vi "ICRA2024最后的ratio控制加轨迹跟踪修改版.vi"() -> ()   [LabVIEW 2018]
doc: "Demonstrates the use of the Network Streams functions to send LED status to the myRIO target."
uses:
  <vilib>/Utility/file.llb/Read Delimited Spreadsheet (string).vi
  <vilib>/ErrorRing/Error Ring.xnode
  <vilib>/vision/NI_Vision_Development_Module.lvlib
panel:
  out "阈值":dbl
  out "ooo":dbl
  out "TT":dbl
  out "与终点距离":sgl
  out "mmm":dbl
  out "期望的ratio":dbl
  out "方向控制量":dbl
  out "速度控制量":dbl
  in  "分裂后的ratio":dbl=3.0
  in  "第二个desiredratio":dbl=7.0
  in  "第一个desiredratio":dbl=3.0
  in  "速度大小":dbl=2.0
  in  "终点纵坐标":dbl=648.0
  in  "终点横坐标":dbl=1450.0
  out "实际纵坐标":sgl[](array[numeric])
  out "实际横坐标":sgl[](array[numeric])
  out "实际纵坐标":sgl
  out "实际横坐标":sgl
  out "方向d1":sgl
  out "轨迹跟踪点数":i32
  out "y":dbl
  out "x":dbl
  out "b":dbl[](array[numeric])
  in  "pp":dbl
  out "与目标点的距离":sgl
  in  "guiji":path=path "D:/lyz/ICRA2024-YuezhenLiu/small_myRIO_Helmholtz - 1111ke777/zgj平滑后的轨迹.txt" caption="call7-8"
  out "ratio误差的绝对值":dbl[](array[numeric])
  in  "pd":dbl=0.1
  out "最终的ratio控制量":dbl
  in  "小p":dbl=1.5
  out "ratio误差的绝对值":dbl
  out "ratio的误差":dbl[](array[numeric])
  out "第二个前馈":dbl
  out "第一个前馈":dbl
  out "后一个ratio误差":dbl
  out "前一个ratio误差":dbl
  out "第一个i":i32
  out "ratio的误差":dbl
  out "裁剪后的二值图":T1(plugin-control)
  in  "布尔":bool
  in  "ribbon磁场开关":bool=TRUE
  out "面积":sgl[](array[numeric])
  out "面积":sgl
  out "数据总":dbl[][](array[numeric])
  out "i":i32[](array[numeric])
  out "aspect ratio":dbl[](array[numeric])
  out "D2":i32[](array[numeric])
  out "D1":i32[](array[numeric])
  out "field ratio":sgl[](array[numeric])
  out "field ratio":sgl=4.0
  out "时间":i32
  in  "打开数据记录":bool
  out "aspect ratio":dbl
  out "D2":i32
  out "D1":i32
  out "二值图":T1(plugin-control)
  in  "Search Rect (entire image)":T2={"Left"=100, "Top"=120, "Right"=2000, "Bottom"=2000, "Rotation"=0.0} {"Rotation" format="%.2f"; "Left" scale=0.0..1024.0; "Right" scale=0.0..1024.0}
  out "备用的椭圆角度":sgl
  in  "Number of Erosion":i32=10
  out "Image 7":T1(plugin-control)
  in  "Acquisition Control::Acquisition Frame Rate":dbl=19.50304412841797 min=1.4211589097976685 max=44.94382095336914
  out "Stopped":bool
  in  "Stop (F) 2":bool caption="Stop (F)"
  out "Objects 2":T3(array[cluster]) {"Aspect Ratio" format="%.2f"; "Orientation" format="%.2f"; "Area" format="%.2f"; "Object Center"."Y" format="%.2f"; "Object Center"."X" format="%.2f"}
  in  "Settings 2":T4={"Objects"=0, "Threshold"=128, "Reject Border"=FALSE, "Fill Holes"=FALSE, "Min Object Size"=FALSE, "Min Size"=20000, "Max Object Size"=FALSE, "Max Size"=100, "Show Search Area"=FALSE, "Show Center"=TRUE, "Show Bounding Box"=TRUE} {"Objects" items=["Bright Objects", "Dark Objects"]; "Threshold" min=1 max=999999999 step=1; "Max Size" min=1 max=999999999 step=1; "Min Size" min=1 max=999999999 step=1}
  in  "Range 2":cluster{"Lower value":sgl, "Upper value":sgl}={"Lower value"=0.0, "Upper value"=230.0} {"Upper value" format="%.2f"; "Lower value" format="%.2f"}
  in  "Pause":bool
  out "Array":dbl[](array[numeric])
  in  "Parameter Settings":T5(tab)=enum."Ribbon Oscillating Field" caption="Field Types"
  in  "fg":dbl
  in  "pg":dbl
  in  "dg":dbl
  in  "Ag":dbl
  in  "AoOF":dbl
  in  "fo":sgl
  in  "do":sgl
  in  "oo":sgl
  in  "po":sgl
  in  "cc":sgl
  in  "pc":sgl
  in  "wc":sgl
  in  "dc":sgl
  in  "Ac":dbl
  in  "pr":sgl
  in  "Ar":dbl=8.0
  in  "wr":sgl=18.0
  in  "dr":sgl
  in  "Dis phase step":dbl
  in  "Dis phase frequency (Hz)":dbl
  in  "Dis tumbling frequency (Hz)":dbl
  in  "Dis strength(mT)":dbl
  in  "Swa strength (mT)":dbl
  in  "Swa frequency (Hz)":dbl
  in  "Swa pitch angle (deg)":dbl
  in  "Swa direction angle (deg)":dbl
  in  "Swa ratio":dbl=1.0
  in  "Pitch Angle (rotating around Constant, deg)":dbl
  in  "Ratio (A/C)":sgl=4.0
  in  "Direction Angle (deg)":sgl
  in  "Pitch Angle (rotating around Origin, deg)":sgl
  in  "Frequency (Hz)":sgl=10.0
  in  "Strength (mT)":dbl=10.0
  in  "Ar 2":dbl=5.0 caption="Ar"
  in  "ratio":sgl=1.0
  in  "运动方向":sgl
  in  "长轴方向":sgl
  in  "wr  2":sgl=8.0
  in  "速度大小":sgl
  out "Numeric 5":i32
  in  "Stop":bool
  out "error out":errorcluster
  in  "Target IP Address":string="172.22.11.2"
  # "Overview: Magnetic field calculation, and send parameters to myRIO\nInstructions:\n1. Verify the value of Target IP Address. Set Visa resource name.\n2. Ensure RT Main.vi is already running. \n3. Run this VI. Set parameters of magnetic field."
  # "Strength (mT)"
  # "Pitch Angle (deg)"
  # "Direction Angle (deg)"
  # "Frequency (Hz)"
  # "Strength (mT)"
  # "Oscilation Frequency (Hz)"
  # "Oscilation Angle (deg)"
  # "Pitch Angle (deg)"
  # "Direction Angle (deg)"
  # "Strength (mT)"
  # "Frequency (Hz)"
  # "Pitch Angle (deg)"
  # "Direction Angle (deg)"
  # "Conical Angle (deg)"
  # "Strength (mT)"
  # "Frequency (Hz)"
  # "Pitch Angle (deg)"
  # "Direction Angle (deg)"
  # "Strength (mT)"
  # "Tumbling Frequency (Hz)"
  # "Phase Frequency (Hz)"
  # "Phase Step"
  # "Strength (mT)"
  # "Frequency (Hz)"
  # "Pitch Angle (deg)"
  # "Direction Angle (deg)"
  # "Ratio"
  # "Strength (mT)"
  # "Frequency (Hz)"
  # "Ratio (A/C)"
  # "Direction Angle (deg)"
  # "Pitch Angle (rotating around Origin, deg)"
  # "Pitch Angle (rotating around Constant, deg)"
  # "Strength (mT)"
  # "Frequency (Hz)"
  # "Pitch Angle  (deg)"
  # "longaxis"
  # "Direction Angle (deg)"
  # "ratio (l/s)"
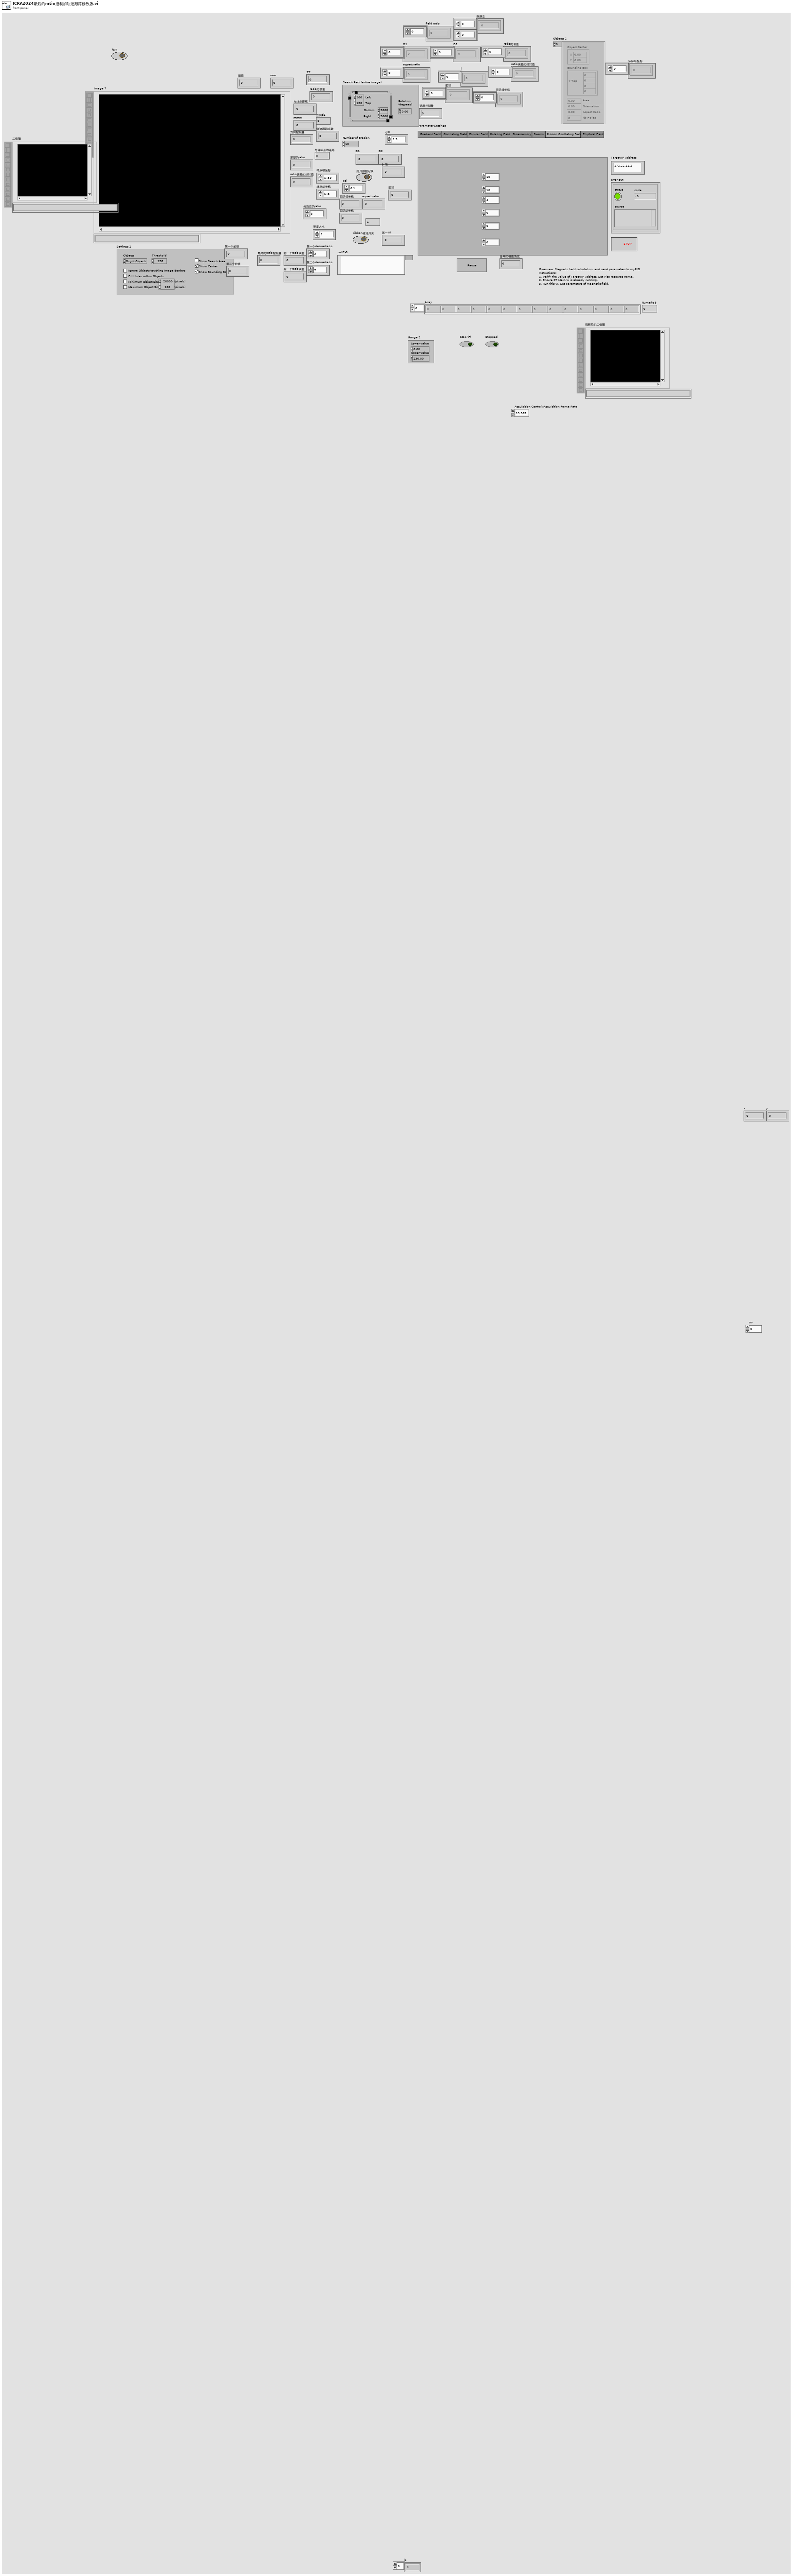
[diagram p1: front panel]
types:
  T1 = typedef "IMAQ Image.ctl" = refnum<image>
  T2 = typedef "IMAQ Rectangle" = cluster{"Left":i32, "Top":i32, "Right":i32, "Bottom":i32, "Rotation":dbl}
  T3 = cluster{"Object Center":cluster{"X":sgl, "Y":sgl}, "Bounding Box":cluster{"X Left":i32, "Y Top":i32, "X Right":i32, "Y Bottom":i32}, "Area":sgl, "Orientation":sgl, "Aspect Ratio":sgl, "Nb Holes":i32}[]
  T4 = cluster{"Objects":u16, "Threshold":i32, "Reject Border":bool, "Fill Holes":bool, "Min Object Size":bool, "Min Size":i32, "Max Object Size":bool, "Max Size":i32, "Show Search Area":bool, "Show Center":bool, "Show Bounding Box":bool}
  T5 = enum32{"Gradient Field ", "Oscillating Field", "Conical Field", "Rotating Field", "Disassembly", "Swarm", "Ribbon Oscillating Field", "Elliptical Field"}
  T6 = typedef "Image Type" = u32
  T7 = cluster{"Objects[0]":cluster{"Object Center":cluster{"X":sgl, "Y":sgl}, "Bounding Box":cluster{"X Left":i32, "Y Top":i32, "X Right":i32, "Y Bottom":i32}, "Area":sgl, "Orientation":sgl, "Aspect Ratio":sgl, "Nb Holes":i32}, "Objects[1]":cluster{"Object Center":cluster{"X":sgl, "Y":sgl}, "Bounding Box":cluster{"X Left":i32, "Y Top":i32, "X Right":i32, "Y Bottom":i32}, "Area":sgl, "Orientation":sgl, "Aspect Ratio":sgl, "Nb Holes":i32}, "Objects[2]":cluster{"Object Center":cluster{"X":sgl, "Y":sgl}, "Bounding Box":cluster{"X Left":i32, "Y Top":i32, "X Right":i32, "Y Bottom":i32}, "Area":sgl, "Orientation":sgl, "Aspect Ratio":sgl, "Nb Holes":i32}, "Objects[3]":cluster{"Object Center":cluster{"X":sgl, "Y":sgl}, "Bounding Box":cluster{"X Left":i32, "Y Top":i32, "X Right":i32, "Y Bottom":i32}, "Area":sgl, "Orientation":sgl, "Aspect Ratio":sgl, "Nb Holes":i32}, "Objects[4]":cluster{"Object Center":cluster{"X":sgl, "Y":sgl}, "Bounding Box":cluster{"X Left":i32, "Y Top":i32, "X Right":i32, "Y Bottom":i32}, "Area":sgl, "Orientation":sgl, "Aspect Ratio":sgl, "Nb Holes":i32}, "Objects[5]":cluster{"Object Center":cluster{"X":sgl, "Y":sgl}, "Bounding Box":cluster{"X Left":i32, "Y Top":i32, "X Right":i32, "Y Bottom":i32}, "Area":sgl, "Orientation":sgl, "Aspect Ratio":sgl, "Nb Holes":i32}, "Objects[6]":cluster{"Object Center":cluster{"X":sgl, "Y":sgl}, "Bounding Box":cluster{"X Left":i32, "Y Top":i32, "X Right":i32, "Y Bottom":i32}, "Area":sgl, "Orientation":sgl, "Aspect Ratio":sgl, "Nb Holes":i32}, "Objects[7]":cluster{"Object Center":cluster{"X":sgl, "Y":sgl}, "Bounding Box":cluster{"X Left":i32, "Y Top":i32, "X Right":i32, "Y Bottom":i32}, "Area":sgl, "Orientation":sgl, "Aspect Ratio":sgl, "Nb Holes":i32}, "Objects[8]":cluster{"Object Center":cluster{"X":sgl, "Y":sgl}, "Bounding Box":cluster{"X Left":i32, "Y Top":i32, "X Right":i32, "Y Bottom":i32}, "Area":sgl, "Orientation":sgl, "Aspect Ratio":sgl, "Nb Holes":i32}}
  T8 = cluster{"Object Center":cluster{"X":sgl, "Y":sgl}, "Bounding Box":cluster{"X Left":i32, "Y Top":i32, "X Right":i32, "Y Bottom":i32}, "Area":sgl, "Orientation":sgl, "Aspect Ratio":sgl, "Nb Holes":i32}
  T9 = cluster{"X Left":i32, "Y Top":i32, "X Right":i32, "Y Bottom":i32}
  T10 = typedef "ROI Descriptor" = cluster{"Global Rectangle":i32[], "Contours":cluster{"ID":enum32{"External", "Internal"}, "Type":u32, "Coordinates":i32[]}[]}
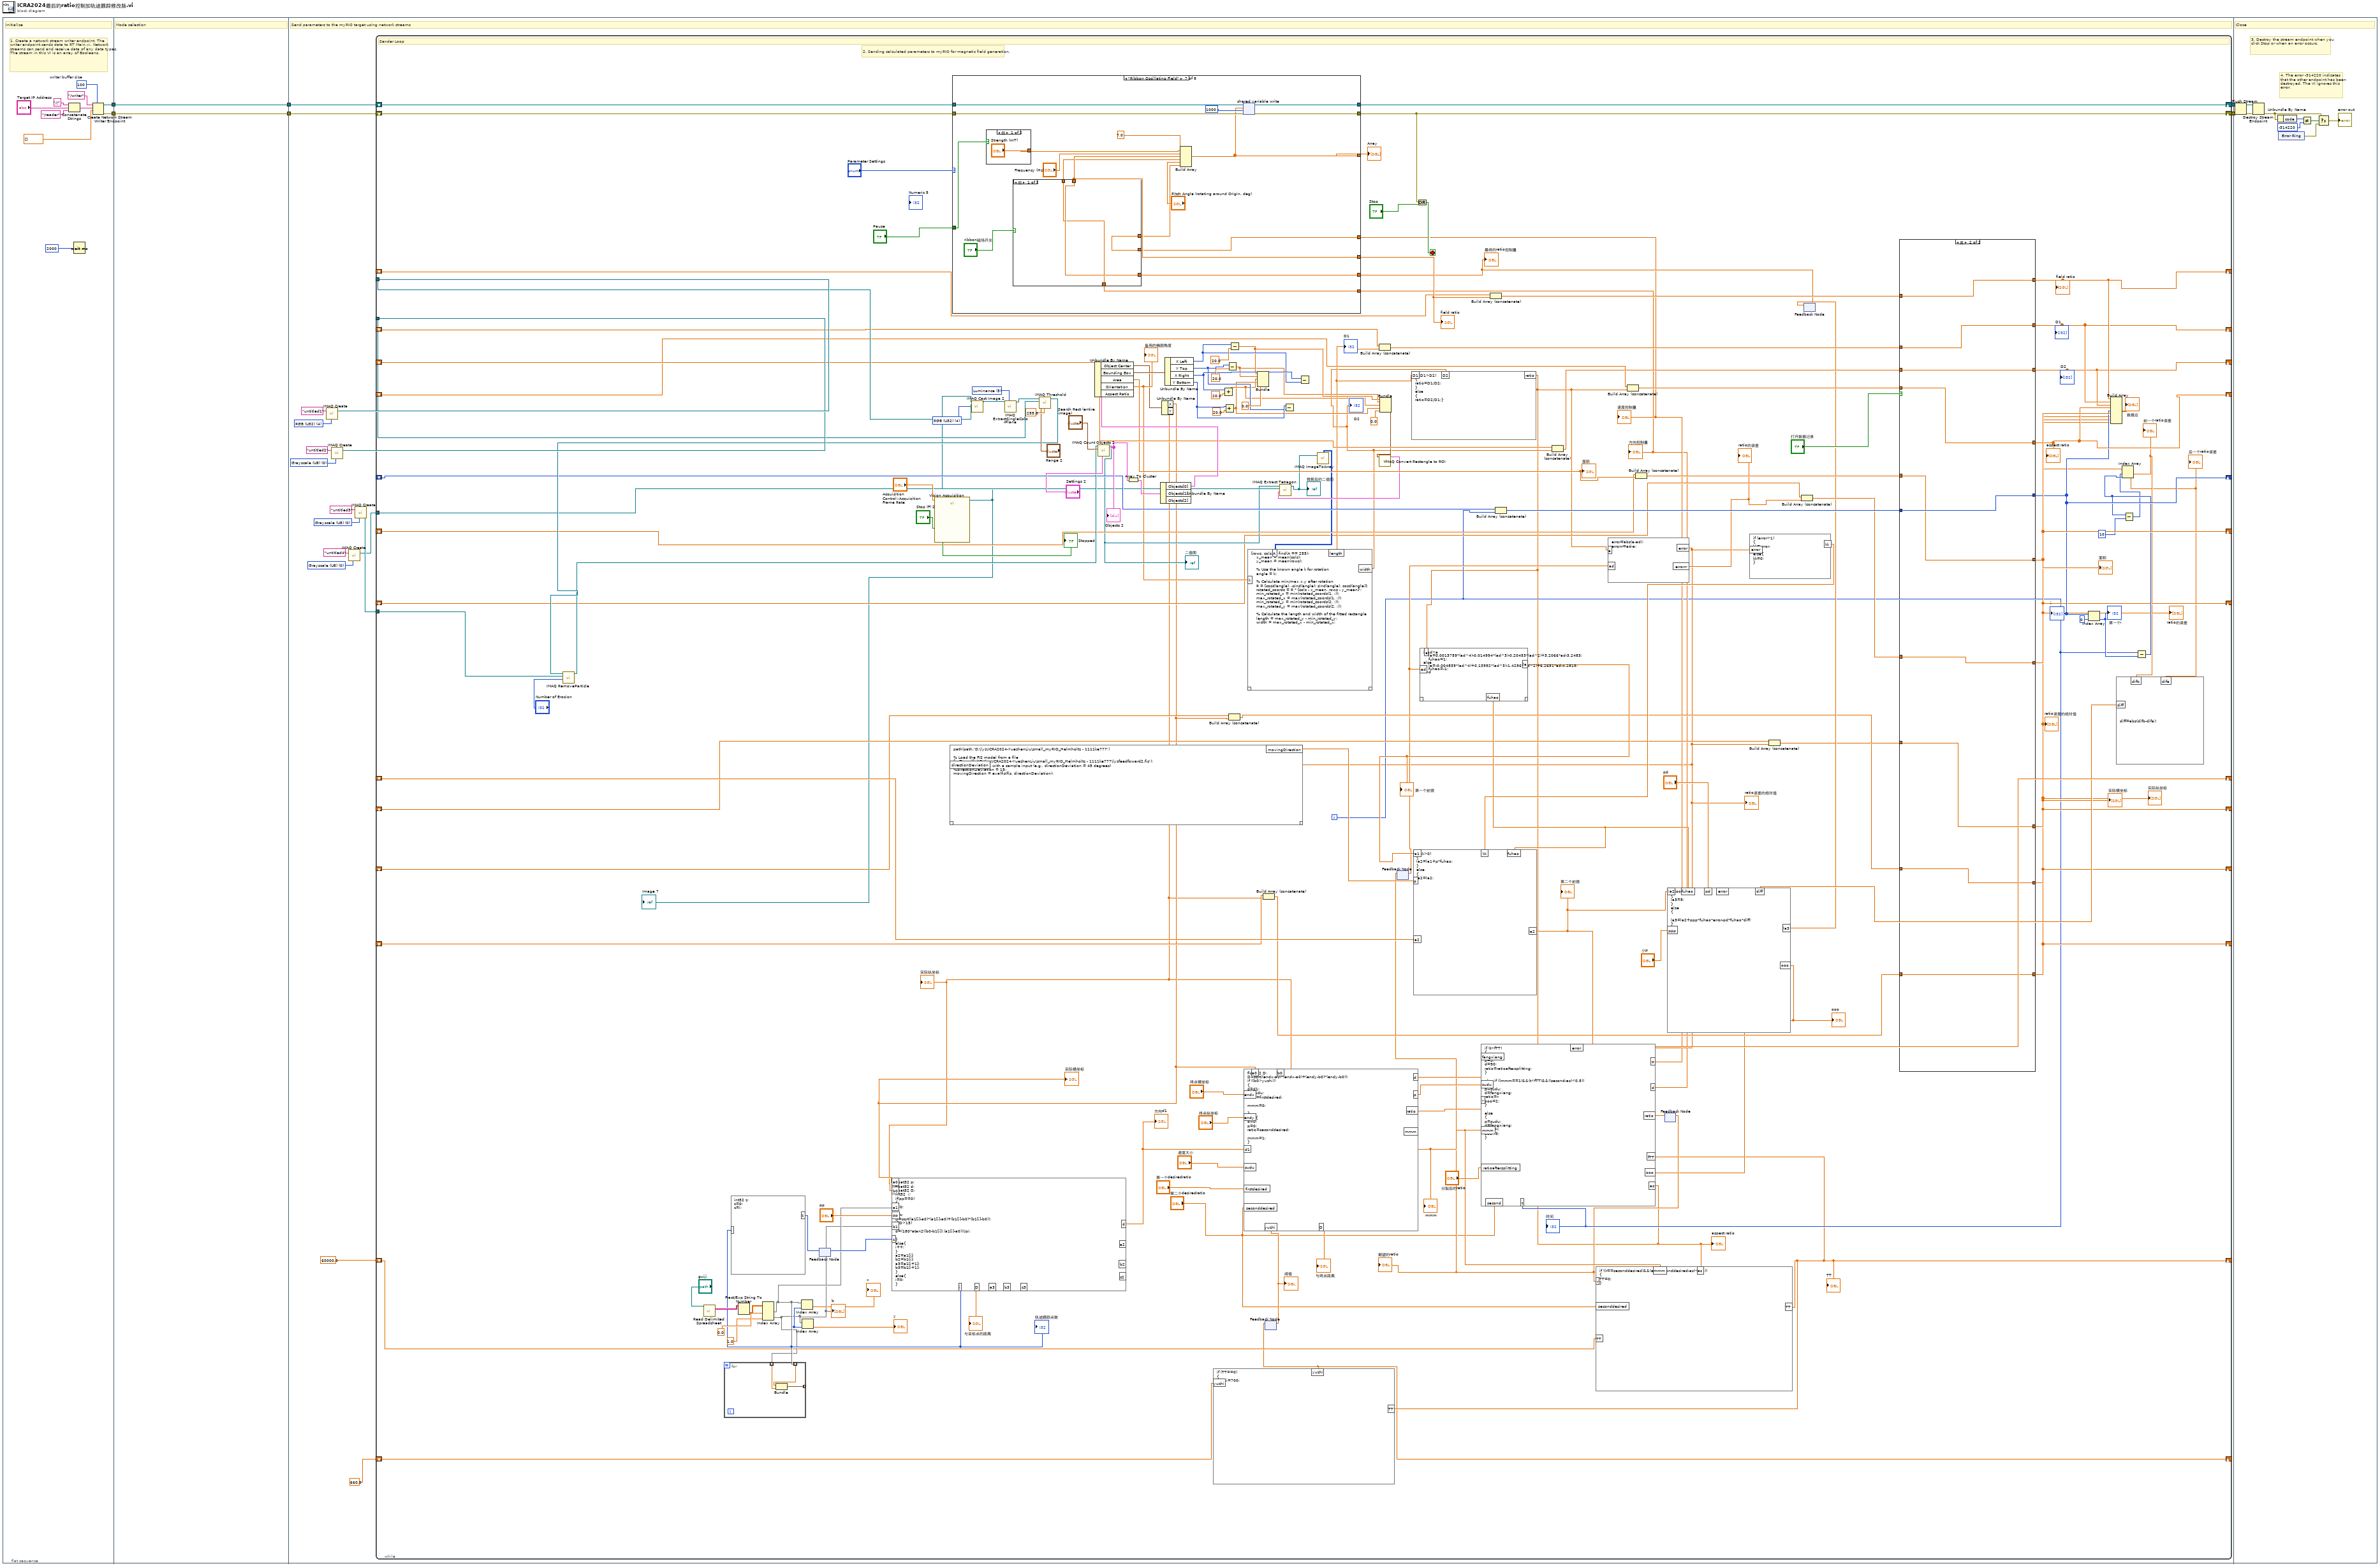
[diagram p0: block diagram]
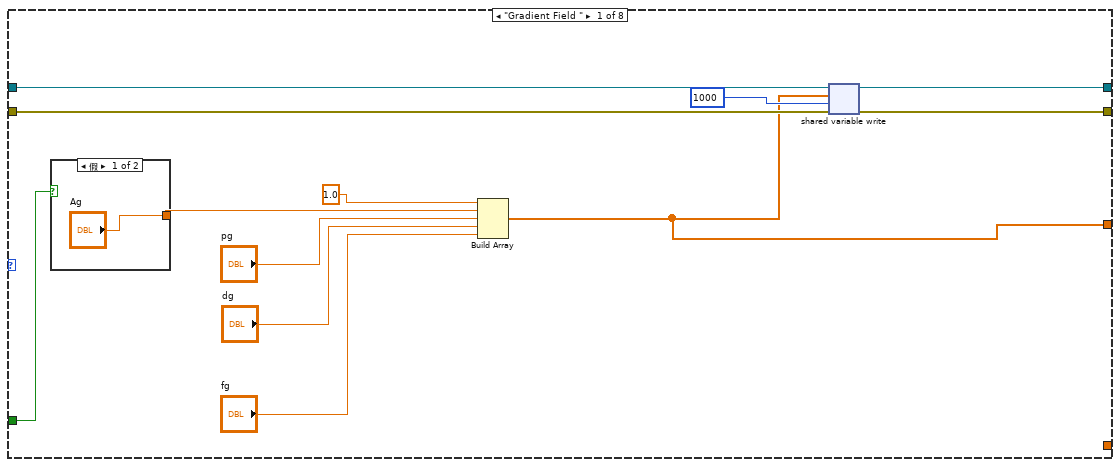
[diagram p3: hidden frame]
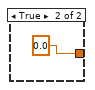
[diagram p4: hidden frame]
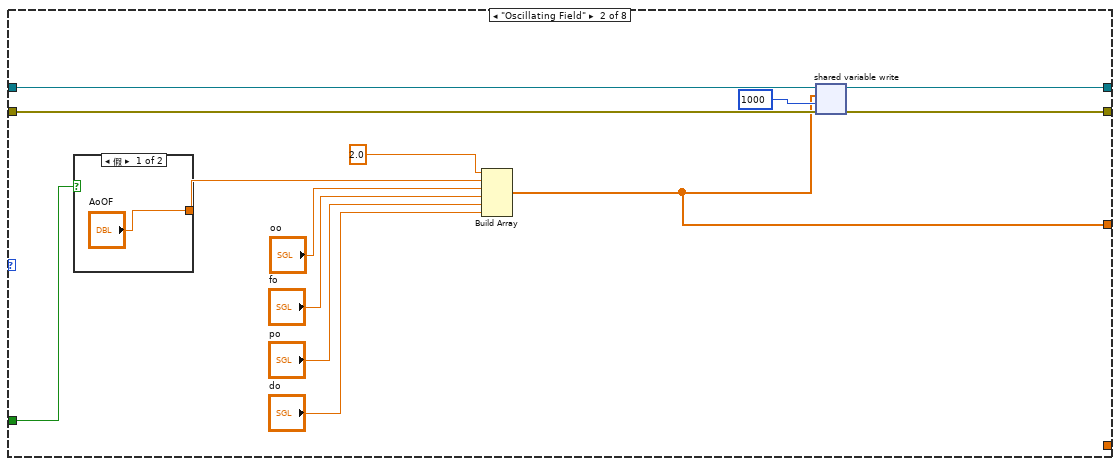
[diagram p5: hidden frame]
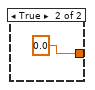
[diagram p6: hidden frame]
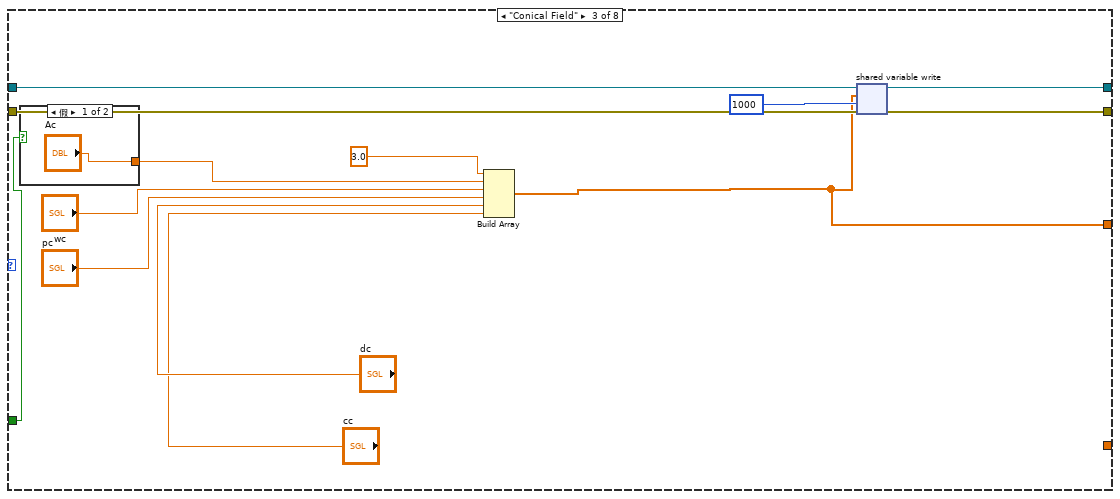
[diagram p7: hidden frame]
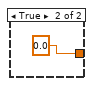
[diagram p8: hidden frame]
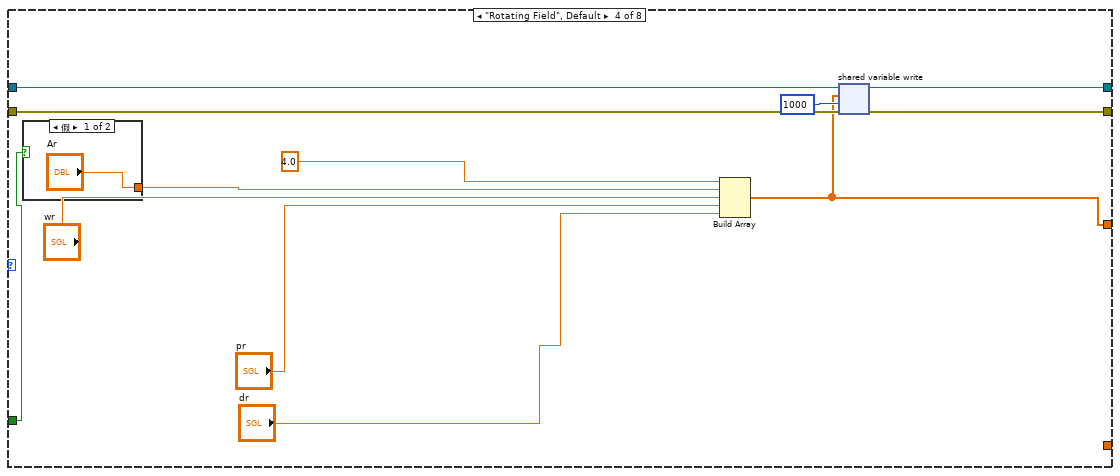
[diagram p9: hidden frame]
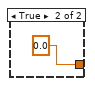
[diagram p10: hidden frame]
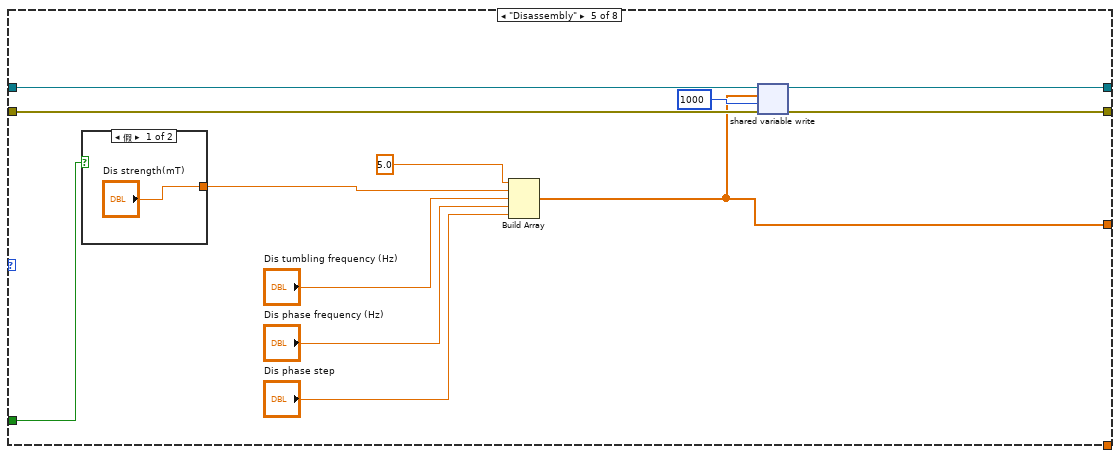
[diagram p11: hidden frame]
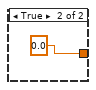
[diagram p12: hidden frame]
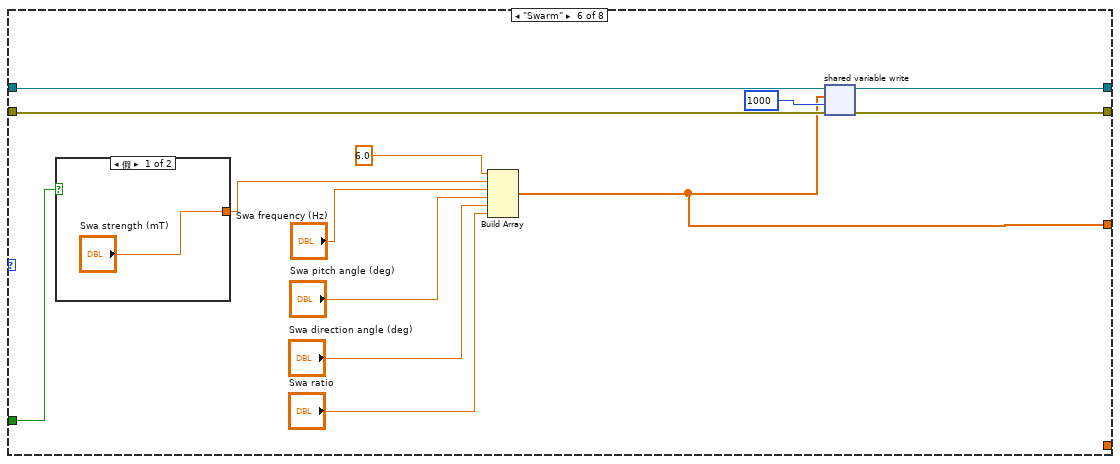
[diagram p13: hidden frame]
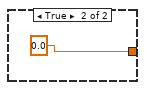
[diagram p14: hidden frame]
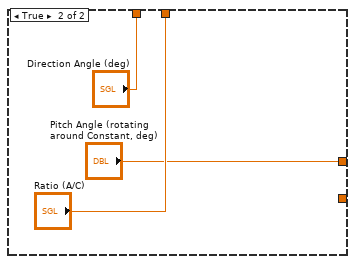
[diagram p15: hidden frame]
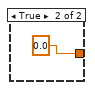
[diagram p16: hidden frame]
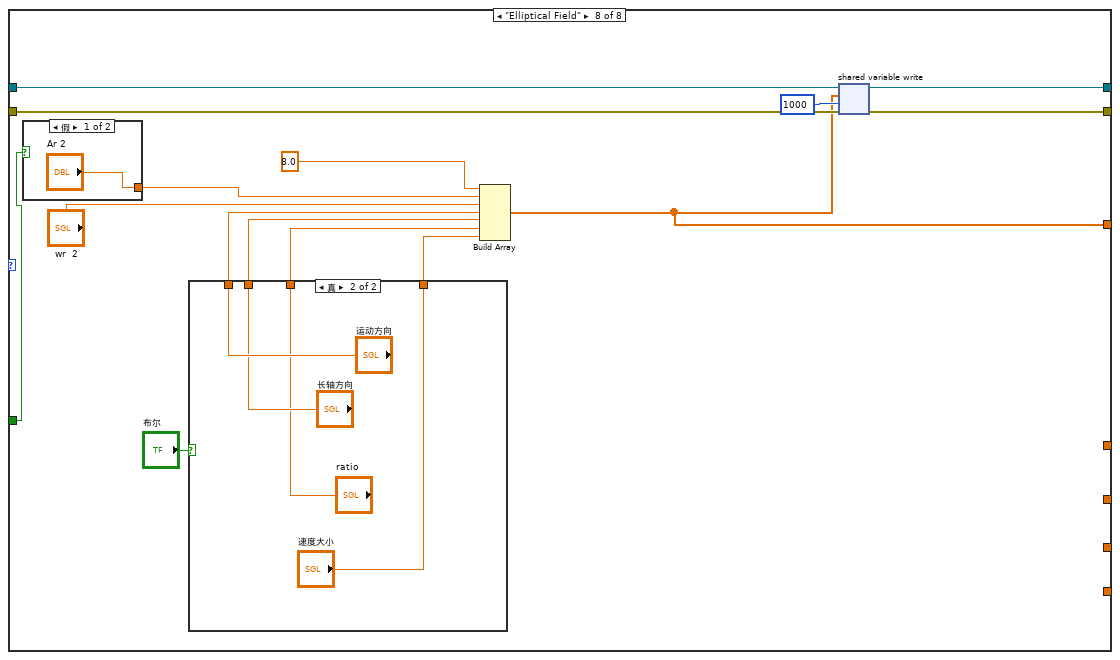
[diagram p17: hidden frame]
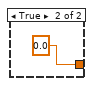
[diagram p19: hidden frame]
diagram:
  n1 = flat-sequence {
    tunnel: [w11] -> w2
    tunnel: [w10] -> w1
    tunnel: [w18] -> w4
    tunnel: [w17] -> w3
    tunnel: w1 -> [w17]
    tunnel: w2 -> [w18]
    tunnel: [w34] -> w6
    tunnel: w4 -> [w36]
    tunnel: [w33] -> w5
    tunnel: w3 -> [w35]
    tunnel: w6 -> [w343]
    tunnel: w5 -> [w340]
    frame #0 {
      w9 = 100  # writer buffer size
      # "1. Create a network stream writer endpoint. The writer endpoint sends data to RT Main.vi. Network streams can send and receive data of any data types. The stream in this VI is an array of Booleans."
      # "Initialize"
      n2 = Concatenate Strings("//", "Target IP Address", "/reader") -> (w16:string)
      n3 = Wait (ms)(milliseconds to wait=2000) -> ()  [unwired: 1 out]
      n4 = Create Network Stream Writer Endpoint(7:w9, 9:dbl[] [], 10:w16, 11:"/writer" ("reader name")) -> (0:w10:errorcluster, 3:w11:refnum<k21>)  [unwired: 3 in]
    }
    frame #1 {
      # "Mode selection"
    }
    frame #2 {
      w22 = T6 0 items=["Grayscale (U8)", "Grayscale (I16)", "Grayscale (SGL)", "Complex (CSG)", "RGB (U32)", "HSL (U32)", "RGB (U64)", "Grayscale (U16)"] ("Image Type")
      w25 = T6 0 items=["Grayscale (U8)", "Grayscale (I16)", "Grayscale (SGL)", "Complex (CSG)", "RGB (U32)", "HSL (U32)", "RGB (U64)", "Grayscale (U16)"] ("Image Type")
      w29 = T6 0 items=["Grayscale (U8)", "Grayscale (I16)", "Grayscale (SGL)", "Complex (CSG)", "RGB (U32)", "HSL (U32)", "RGB (U64)", "Grayscale (U16)"] ("Image Type")
      w31 = T6 4 items=["Grayscale (U8)", "Grayscale (I16)", "Grayscale (SGL)", "Complex (CSG)", "RGB (U32)", "HSL (U32)", "RGB (U64)", "Grayscale (U16)"] ("Image Type")
      # "Send parameters to the myRIO target using network streams"
      n5 = call "IMAQ Create"("Image Name"="untitled1", "Image Type"=w31) -> ("New Image"=w28:T1)  [unwired: 3 in, 1 out]
      n6 = call "IMAQ Create"("Image Name"="untitled2", "Image Type"=w29) -> ("New Image"=w27:T1)  [unwired: 3 in, 1 out]
      n7 = call "IMAQ Create"("Image Name"="untitled4", "Image Type"=w22) -> ("New Image"=w21:T1)  [unwired: 3 in, 1 out]
      n8 = call "IMAQ Create"("Image Name"="untitled3", "Image Type"=w25) -> ("New Image"=w24:T1)  [unwired: 3 in, 1 out]
      n9 = while {
        shift-right: [w182] -> w33
        shift-left: w35 -> [w184]
        shift-right: [w183] -> w34
        shift-left: w36 -> [w185]
        tunnel: w27 -> [w173]
        tunnel: w28 -> [w168]
        tunnel: w24 -> [w157]
        shift-right: [w135] -> _
        shift-left: _ -> [w144]
        shift-right: [w134] -> _
        shift-left: _ -> [w142]
        shift-right: [w133] -> _
        shift-left: _ -> [w140]
        shift-right: [w114] -> _
        shift-left: _ -> [w138]
        shift-right: [w113] -> _
        shift-left: _ -> [w136]
        shift-right: [w129] -> _
        shift-left: _ -> [w128]
        tunnel: w21 -> [w127]
        shift-right: [w104] -> _
        shift-left: _ -> [w105]
        shift-right: [w102] -> _
        shift-left: _ -> [w101]
        shift-right: [w87] -> _
        shift-left: _ -> [w88]
        shift-right: [w66] -> _
        shift-left: _ -> [w69]
        shift-right: [w65] -> _
        shift-left: _ -> [w67]
        shift-right: [w42] -> _
        shift-left: 60000.0 -> [w49]
        shift-right: [w40] -> _
        shift-left: 660.0 -> [w39]
        i -> [w50]
        stop <- w172 stop-if-true
        w167 = T6 4 items=["Grayscale (U8)", "Grayscale (I16)", "Grayscale (SGL)", "Complex (CSG)", "RGB (U32)", "HSL (U32)", "RGB (U64)", "Grayscale (U16)"] ("Image Type")
        w178 = 5 items=["Red", "Green", "Blue", "Hue", "Saturation", "Luminance", "Value", "Intensity"] ("Color Plane")
        # "2. Sending calculated parameters to myRIO for magnetic field generation."
        # "Sender Loop"
        n10 = call-poly <vilib>:"Read Delimited Spreadsheet.vi"("file path (dialog if empty)"="guiji") -> ("all rows"=w84:string[][])  [unwired: 9 in, 5 out]
        n11 = Fract/Exp String To Number(string=w84) -> (number=w83:dbl[][])  [unwired: 3 in, 1 out]
        n12 = Index Array(array=w83, index (col) #1=0.0, index (col) #2=1.0) -> (element #1=w76:dbl[], element #2=w74:dbl[])  [unwired: 2 in]
        "b" <- w74
        n13 = for {
          tunnel: w76 -> [w189] mode=indexing
          tunnel: w74 -> [w188] mode=indexing
          tunnel: [w187] -> _ mode=indexing
          n14 = Bundle("String"=w189, "String"=w188) -> (w187:cluster{"String":dbl, "String":dbl})  [unwired: 1 in]
        }
        n15 = feedback #1() -> (w79:i32)  [unwired: 1 in]
        n16 = call "Vision Acquisition"("Acquisition Control::Acquisition Frame Rate"="Acquisition Control::Acquisition Frame Rate", "Stop (F)"="Stop (F) 2") -> ("Image Out"=w86:T1, "Stopped"=→"Stopped":bool)  [unwired: 23 in, 1 out]
        "Image 7" <- w86
        n17 = call "IMAQ Cast Image 2"("Image Src"=w86, "Image Dst"=w168, "Image Type"=w167) -> ("Image Dst Out"=w169:T1)  [unwired: 11 in, 1 out]
        n18 = call "IMAQ ExtractSingleColorPlane"("Color Plane"=w178, "Image Src"=w169) -> ("Image Dst Out"=w155:T1)  [unwired: 8 in, 1 out]
        n19 = call "IMAQ Threshold"("Replace Value"=sgl 255.0, "Range"="Range 2", "Image Dst"=w173, "Image Src"=w155) -> ("Image Dst Out"=w158:T1)  [unwired: 6 in, 1 out]
        n20 = call "IMAQ RemoveParticle"("Number of Erosion"="Number of Erosion", "Image Dst"=w157, "Image Src"=w158) -> ("Image Dst Out"=w150:T1)  [unwired: 7 in, 1 out]
        n21 = call "IMAQ Count Objects 2"("Settings"="Settings 2", "Search Rect (entire image)"="Search Rect (entire image)", "Image"=w150) -> ("Image Out"=w126:T1, "Objects"=w174:T3)  [unwired: 4 in, 3 out]
        "Objects 2" <- w174
        "二值图" <- w126
        n22 = Array To Cluster(array=w174) -> (cluster=w160:T7)
        n23 = Unbundle By Name(w160) -> ("Objects[0]"=w159:T8)  [unwired: 2 out]
        n24 = Unbundle By Name(w159) -> ("Object Center"=w71:cluster{"X":sgl, "Y":sgl}, "Bounding Box"=w166:T9, "Area"=w131:sgl, "Orientation"=w110:sgl)  [unwired: 1 out]
        "备用的椭圆角度" <- w110
        "面积" <- w131
        n25 = Unbundle By Name(w71) -> ("X"=w60:sgl, "Y"=w59:sgl)
        "实际横坐标" <- w60
        "实际纵坐标" <- w59
        n26 = formula code="float32 p;\nfloat32 d;\nfloat32 D;\nint32  i;\nif(pp==0)\n{\ni=0;\n\ni=z;\nD=sqrt((a1[i]-a0)*(a1[i]-a0)+(b1[i]-b0)*(b1[i]-b0));\nif(D>15)\n{\nd=(180*atan2((b0-b1[i]),(a1[i]-a0)))/pi;\n\n}\nelse{\ni++;\n}\na2=a1[i];\nb2=b1[i];\na3=a1[i+1];\nb3=b1[i+1];\n}\nelse{\ni=0;\n}"("a0"=w60, "b0"=w59, "a1"=w76, "b1"=w74, "z"=w79, "pp"="pp") -> ("i"=w75:i32, "D"=→"与目标点的距离":sgl, "d"=w62:sgl)  [unwired: 6 out]
        "轨迹跟踪点数" <- w75
        "方向d1" <- w62
        n27 = formula code="int32 z;\nz=0;\nz=i;"("i"=w75) -> ("z"=w80:i32)
        n28 = Index Array(array=w76, index=w75) -> (element=→"x":dbl)
        n29 = Index Array(array=w74, index=w75) -> (element=→"y":dbl)
        n30 = feedback-in #1(w80) -> ()
        n31 = Unbundle By Name(w166) -> ("X Left"=w152:i32, "Y Top"=w148:i32, "X Right"=w153:i32, "Y Bottom"=w149:i32)
        n32 = Add(x=w153, y=20.0) -> (x+y=w121:dbl)
        n33 = Add(x=w149, y=20.0) -> (x+y=w120:dbl)
        n34 = Subtract(x=w148, y=20.0) -> (x-y=w122:dbl)
        n35 = Build Array (concatenate)(w69, w60) -> (w70:sgl[])
        n36 = Subtract(x=w152, y=20.0) -> (x-y=w123:dbl)
        n37 = Bundle(w123, w122, w121, w120, 0.0) -> ()  [unwired: 1 in, 1 out]
        n38 = Build Array (concatenate)(w67, w59) -> (w68:sgl[])
        n39 = feedback #2() -> (w41:dbl)  [unwired: 1 in]
        "阈值" <- w41
        n40 = formula code="float32 D;\nD=sqrt((endx-a0)*(endx-a0)+(endy-b0)*(endy-b0));\nif ((b0>yuzhi))\n{\nd=d1;\np=sudu;\nratio=firstdesired;\n\nmmm=0;\n\n}\nelse{\nd=0;\np=0;\nratio=seconddesired;\n\nmmm=1;\n}"("endx"="终点横坐标", "endy"="终点纵坐标", "d1"=w62, "sudu"="速度大小", "firstdesired"="第一个desiredratio", "seconddesired"="第二个desiredratio", "a0"=w60, "b0"=w59, "yuzhi"=w41) -> ("p"=w57:dbl, "ratio"=w46:dbl, "d"=w56:dbl, "mmm"=w47:dbl, "D"=→"与终点距离":sgl)
        "mmm" <- w47
        n41 = Subtract(x=w149, y=w148) -> ()  [unwired: 1 out]
        n42 = Subtract(x=w153, y=w152) -> ()  [unwired: 1 out]
        n43 = Bundle(w123, w122, w121, w120, 0.0) -> (w118:cluster{dbl, dbl, dbl, dbl, dbl})  [unwired: 1 in]
        n44 = call "IMAQ Convert Rectangle to ROI"("Rectangle"=w118) -> ("ROI Descriptor"=w124:T10)  [unwired: 8 in, 1 out]
        n45 = call-poly "IMAQ Extract Tetragon"("ROI Descriptor"=w124, "Image Dst"=w127, "Image Src"=w126) -> ("Image Dst Out"=w125:T1)  [unwired: 7 in, 1 out]
        "裁剪后的二值图" <- w125
        n46 = call "IMAQ ImageToArray"("Image"=w125) -> ("Image Pixels (U8)"=w117:u8[][])  [unwired: 3 in, 4 out]
        n47 = script code="[rows, cols] = find(A == 255);\n    x_mean = mean(cols);\n    y_mean = mean(rows);\n\n    % Use the known angle k for rotation\n    angle = k;\n\n    % Calculate min/max x,y after rotation\n    R = [cosd(angle), -sind(angle); sind(angle), cosd(angle)];\n    rotated_coords = R * [cols - x_mean, rows - y_mean]';\n    min_rotated_x = min(rotated_coords(1, :));\n    max_rotated_x = max(rotated_coords(1, :));\n    min_rotated_y = min(rotated_coords(2, :));\n    max_rotated_y = max(rotated_coords(2, :));\n\n    % Calculate the length and width of the fitted rectangle\n    length = max_rotated_y - min_rotated_y;\n    width = max_rotated_x - min_rotated_x;"("A"=w117, "k"=w110) -> ("length"=w116:dbl, "width"=w115:dbl)  [unwired: 1 in, 1 out]
        "D1" <- w116
        "D2" <- w115
        n48 = Build Array (concatenate)(w142, w116) -> (w143:dbl[])
        n49 = feedback #3() -> (w54:dbl)  [unwired: 1 in]
        n50 = formula code="if (D1>D2)\n{\nratio=D1/D2;\n}\nelse\n{\nratio=D2/D1;}"("D1"=w116, "D2"=w115) -> ("ratio"=w38:dbl)
        "aspect ratio" <- w38
        n51 = script code="if ad>a\n    la=0.0013759*(ad^4)-0.014994*(ad^3)-0.20453*(ad^2)+3.2066*ad-3.2483;\n    fuhao=1;\nelse\n    la=-0.004839*(ad^4)+0.13992*(ad^3)-1.4256*(ad^2)+6.2651*ad-4.2815;\n    fuhao=-1;\nend"("a"=w38, "ad"=w54) -> ("la"=w92:dbl, "fuhao"=w91:dbl)  [unwired: 1 in, 1 out]
        "第一个前馈" <- w92
        n52 = Build Array (concatenate)(w136, w50) -> (w137:i32[])
        n53 = Build Array (concatenate)(w140, w115) -> (w141:dbl[])
        n54 = formula code="error=abs(a-ad);\nerrorrr=ad-a;"("a"=w38, "ad"=w54) -> ("error"=w48:dbl, "errorrr"=w97:dbl)
        "ratio的误差" <- w97
        "ratio误差的绝对值" <- w48
        n55 = script code="path(path,'D:\\lyz\\ICRA2024-YuezhenLiu\\small_myRIO_Helmholtz - 1111ke777')\n\n% Load the FIS model from a file\nfis = readfis('D:\\lyz\\ICRA2024-YuezhenLiu\\small_myRIO_Helmholtz - 1111ke777\\lyzfeedfoward2.fis');\n% Evaluate the FIS with a sample input (e.g., directionDeviation = 45 degrees)\n%directionDeviation = 15;\nmovingDirection = evalfis(fis, directionDeviation);"("directionDeviation"=w48) -> ("movingDirection"=w90:dbl)  [unwired: 1 in, 1 out]
        n56 = Build Array (concatenate)(w138, w38) -> (w139:dbl[])
        n57 = Build Array (concatenate)(w128, w131) -> (w130:sgl[])
        n58 = feedback #4() -> (w44:dbl)  [unwired: 1 in]
        "期望的ratio" <- w44
        n59 = feedback-in #3(w44) -> ()
        n60 = formula code="if ((r==seconddesired)&&(abs(seconddesired-as)<0.5))\n{\nTT=0;\n}"("TT"=w49, "mmm"=w47, "as"=w38, "r"=w44, "seconddesired"="第二个desiredratio") -> ("TT"=w42:dbl)
        "TT" <- w42
        n61 = formula code="if (TT==0)\n{\nyuzhi=700;\n}"("TT"=w42, "yuzhi"=w39) -> ("yuzhi"=w40:dbl)
        n62 = feedback-in #2(w40) -> ()
        n63 = formula code="if (t>fTT)\n{\nooo=1;\np=3;\nd=90;\nratio=ratioaftersplitting;\n}\n\nelse if ((mmm==1)&&(t<fTT)&&((second-as)<0.5))\n{\np=sudu;\nd=fangxiang;\nratio=r;\nooo=2;\n}\n\nelse\n{\np=sudu;\nd=fangxiang;\nratio=r;\nooo=3;\n}"("mmm"=w47, "sudu"=w57, "fangxiang"=w56, "r"=w46, "error"=w48, "ratioaftersplitting"="分裂后的ratio", "t"=w50, "fTT"=w42, "as"=w38, "second"="第二个desiredratio") -> ("p"=w53:dbl, "d"=w52:dbl, "ratio"=w45:dbl, "ooo"=w43:dbl)
        "速度控制量" <- w53
        "方向控制量" <- w52
        "ooo" <- w43
        n64 = feedback-in #4(w45) -> ()
        n65 = formula code="if (error>1)\n{\nkk=error;\n}\nelse{\nkk=0;\n}"("error"=w48) -> ("kk"=w106:dbl)
        n66 = formula code="if(kk>0)\n{\nla2=la1+p*fuhao;\n}\nelse\n{\nla2=la2;\n}"("kk"=w106, "la1"=w92, "fuhao"=w91, "p"=w90, "la2"=w105) -> ("la2"=w104:dbl)
        "第二个前馈" <- w104
        n67 = Build Array (concatenate)(w88, w48) -> (w89:dbl[])
        n68 = Build Array (concatenate)(w101, w97) -> (w103:dbl[])
        n69 = feedback #5() -> (w94:dbl)  [unwired: 1 in]
        "最终的ratio控制量" <- w94
        n70 = case shown="\"Ribbon Oscillating Field\"" "Parameter Settings" {
          tunnel: w185 -> [w210 w225 w240 w254 w268 w282 w304 w326]
          tunnel: w184 -> [w207 w224 w239 w253 w266 w281 w302 w325]
          tunnel: [w209 w223 w237 w252 w267 w280 w303 w324] -> w183
          tunnel: [w208 w222 w238 w251 w265 w279 w301 w323] -> w182
          tunnel: [w203 w216 w231 w246 w259 w274 w299 w318] -> w181
          tunnel: "Pause" -> [w201 w214 w229 w244 w258 w273 w296 w316]
          tunnel: [_ _ _ _ _ _ w294 _] -> w146
          tunnel: w94 -> [_ _ _ _ _ _ w291 _]
          tunnel: w53 -> [_ _ _ _ _ _ w288 _]
          tunnel: w52 -> [_ _ _ _ _ _ w287 _]
          frame "Gradient Field " {
            n71 = case shown="假" w201 {
              tunnel: ["Ag" 0.0] -> w202
              frame False {
              }
              frame True {
              }
            }
            n72 = Build Array(1.0, w202, "pg", "dg", "fg") -> (w203:dbl[])
            n73 = shared-variable-write(w210, w207, w203, 1000 ("timeout ms (-1)")) -> (w209:refnum<k21>, w208:errorcluster)  [unwired: 1 out]
          }
          frame "Oscillating Field" {
            n74 = case shown="假" w214 {
              tunnel: ["AoOF" 0.0] -> w215
              frame False {
              }
              frame True {
              }
            }
            n75 = Build Array(2.0, w215, "oo", "fo", "po", "do") -> (w216:dbl[])
            n76 = shared-variable-write(w225, w224, w216, 1000 ("timeout ms (-1)")) -> (w223:refnum<k21>, w222:errorcluster)  [unwired: 1 out]
          }
          frame "Conical Field" {
            # "FG"
            n77 = case shown="假" w229 {
              tunnel: ["Ac" 0.0] -> w230
              frame False {
              }
              frame True {
              }
            }
            n78 = Build Array(3.0, w230, "wc", "pc", "dc", "cc") -> (w231:dbl[])
            n79 = shared-variable-write(w240, w239, w231, 1000 ("timeout ms (-1)")) -> (w237:refnum<k21>, w238:errorcluster)  [unwired: 1 out]
          }
          frame "Rotating Field", Default {
            n80 = case shown="假" w244 {
              tunnel: ["Ar" 0.0] -> w245
              frame False {
              }
              frame True {
              }
            }
            n81 = Build Array(4.0, w245, "wr", "pr", "dr") -> (w246:dbl[])
            n82 = shared-variable-write(w254, w253, w246, 1000 ("timeout ms (-1)")) -> (w252:refnum<k21>, w251:errorcluster)  [unwired: 1 out]
          }
          frame "Disassembly" {
            n83 = case shown="假" w258 {
              tunnel: ["Dis strength(mT)" 0.0] -> w263
              frame False {
              }
              frame True {
              }
            }
            n84 = Build Array(5.0, w263, "Dis tumbling frequency (Hz)", "Dis phase frequency (Hz)", "Dis phase step") -> (w259:dbl[])
            n85 = shared-variable-write(w268, w266, w259, 1000 ("timeout ms (-1)")) -> (w267:refnum<k21>, w265:errorcluster)  [unwired: 1 out]
          }
          frame "Swarm" {
            n86 = case shown="假" w273 {
              tunnel: ["Swa strength (mT)" 0.0] -> w272
              frame False {
              }
              frame True {
              }
            }
            n87 = Build Array(6.0, w272, "Swa frequency (Hz)", "Swa pitch angle (deg)", "Swa direction angle (deg)", "Swa ratio") -> (w274:dbl[])
            n88 = shared-variable-write(w282, w281, w274, 1000 ("timeout ms (-1)")) -> (w280:refnum<k21>, w279:errorcluster)  [unwired: 1 out]
          }
          frame "Ribbon Oscillating Field" {
            n89 = case shown="假" w296 {
              tunnel: ["Strength (mT)" 0.0] -> w295
              frame False {
              }
              frame True {
              }
            }
            n90 = case shown="假" "ribbon磁场开关" {
              tunnel: [w307 "Ratio (A/C)"] -> w294
              tunnel: w291 -> [w307 _]
              tunnel: [w305 "Direction Angle (deg)"] -> w290
              tunnel: [w306 "Pitch Angle (rotating around Constant, deg)"] -> w289
              tunnel: w288 -> [w306 _]
              tunnel: w287 -> [w305 _]
              frame False {
              }
              frame True {
              }
            }
            n91 = Build Array(7.0, w295, "Frequency (Hz)", w294, w290, "Pitch Angle (rotating around Origin, deg)", w289) -> (w299:dbl[])
            n92 = shared-variable-write(w304, w302, w299, 1000 ("timeout ms (-1)")) -> (w303:refnum<k21>, w301:errorcluster)  [unwired: 1 out]
          }
          frame "Elliptical Field" {
            n93 = case shown="假" w316 {
              tunnel: ["Ar 2" 0.0] -> w317
              frame False {
              }
              frame True {
              }
            }
            n94 = case shown="真" "布尔" {
              tunnel: [_ "运动方向"] -> w321
              tunnel: [_ "长轴方向"] -> w320
              tunnel: [_ "ratio"] -> w315
              tunnel: [_ "速度大小"] -> w314
              frame False {
              }
              frame True {
              }
            }
            n95 = Build Array(8.0, w317, "wr  2", w321, w320, w315, w314) -> (w318:dbl[])
            n96 = shared-variable-write(w326, w325, w318, 1000 ("timeout ms (-1)")) -> (w324:refnum<k21>, w323:errorcluster)  [unwired: 1 out]
          }
        }
        "Array" <- w181
        "field ratio" <- w146
        n97 = Or(x=w182, y="Stop") -> (x .or. y?=w172:bool)
        n98 = Build Array (concatenate)(w144, w146) -> (w145:dbl[])
        n99 = case shown="真" "打开数据记录" {
          tunnel: [_ w199] -> w135
          tunnel: w145 -> [_ w199]
          tunnel: [_ w198] -> w134
          tunnel: w143 -> [_ w198]
          tunnel: [_ w197] -> w133
          tunnel: w141 -> [_ w197]
          tunnel: [_ w196] -> w114
          tunnel: w139 -> [_ w196]
          tunnel: [_ w195] -> w113
          tunnel: w137 -> [_ w195]
          tunnel: [_ w194] -> w129
          tunnel: w130 -> [_ w194]
          tunnel: [_ w193] -> w102
          tunnel: w103 -> [_ w193]
          tunnel: [_ w192] -> w87
          tunnel: w89 -> [_ w192]
          tunnel: [_ w191] -> w66
          tunnel: w70 -> [_ w191]
          tunnel: [_ w190] -> w65
          tunnel: w68 -> [_ w190]
          frame False {
          }
          frame True {
          }
        }
        "field ratio" <- w135
        "D1" <- w134
        "D2" <- w133
        "aspect ratio" <- w114
        "i" <- w113
        "面积" <- w129
        "ratio的误差" <- w102
        "ratio误差的绝对值" <- w87
        "实际横坐标" <- w66
        "实际纵坐标" <- w65
        n100 = Index Array(array=w113, index=0 ("索引")) -> (element=w111:i32)
        "第一个i" <- w111
        n101 = Build Array(w135, w134, w133, w114, w113, w129, w87, w66, w65) -> (→"数据总":dbl[][])
        n102 = Subtract(x=w50, y=w111) -> (x-y=w109:i32)
        n103 = Subtract(x=w109, y=10) -> (x-y=w108:i32)
        n104 = Index Array(array=w102, index #1=w108, index #2=w109) -> (element #1=w100:dbl, element #2=w99:dbl)
        "前一个ratio误差" <- w100
        "后一个ratio误差" <- w99
        n105 = formula code="diff=abs(difb-difa);"("difb"=w100, "difa"=w99) -> ("diff"=w98:dbl)
        n106 = formula code="if (ooo==1)\n{\nla3=5;\n}\nelse\n{\n\nla3=la2+ppp*fuhao*error-pd*fuhao*diff;\n}"("la2"=w104, "fuhao"=w91, "diff"=w98, "ppp"="小p", "pd"="pd", "error"=w48, "ooo"=w43) -> ("la3"=w95:dbl)
        n107 = feedback-in #5(w95) -> ()
        "时间" <- w50
      }
    }
    frame #3 {
      # "4. The error -314220 indicates that the other endpoint has been destroyed. The VI ignores this error."
      # "3. Destroy the stream endpoint when you click Stop or when an error occurs."
      # "Close"
      n108 = Flush Stream(8:w340, 11:w343) -> (0:w341:errorcluster, 3:w342:refnum<k21>)  [unwired: 2 in, 1 out]
      n109 = Destroy Stream Endpoint(8:w341, 11:w342) -> (0:w335:errorcluster)
      n110 = Unbundle By Name(w335) -> ("code"=w339:i32)
      n111 = xnode "Error Ring"() -> ("错误输出"=w336:errorcluster)
      n112 = Not Equal?(x=w339, y=-314220) -> (x != y?=w337:bool)
      n113 = Select(t=w335, s=w337, f=w336) -> (s? t:f=→"error out":errorcluster)
    }
  }
